vi "Bitfile.Initialize.vi"(8 "error in (no error)":errorcluster, 11 "FPGA Bitfile Settings":T1) -> (0 "error out":errorcluster, 3 "FPGA Session":u32)   [LabVIEW 2019, in "Diagnostics Addon Engine.lvlib"]
uses:
  Diagnostics Addon Engine.lvlib
  Addon Shared/Types/986x.ctl
  Addon Shared/Diagnostics Addon Shared.lvlib
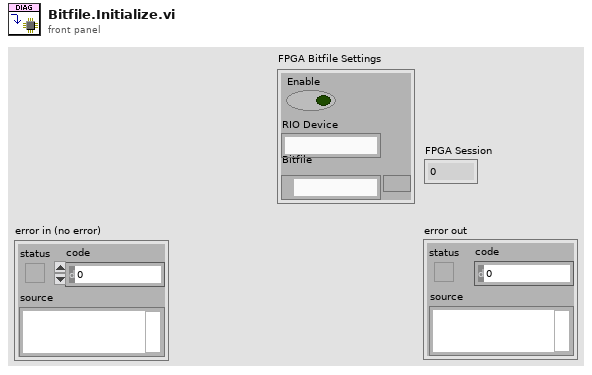
[diagram p1: front panel]
types:
  T1 = typedef "Diagnostics Addon Shared.lvlib/986x.ctl" = cluster{"Enable":bool, "RIO Device":string, "Bitfile":path}
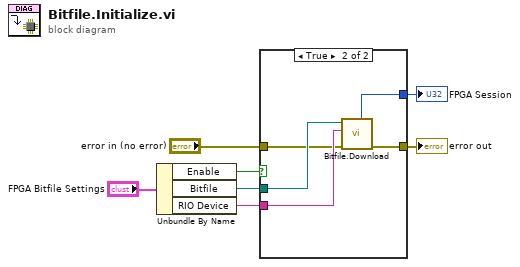
[diagram p0: block diagram]
diagram:
  n1 = Unbundle By Name("FPGA Bitfile Settings") -> ("Enable"=w3:bool, "Bitfile"=w2:path, "RIO Device"=w4:string)
  n2 = case shown="True" w3 {
    tunnel: "error in (no error)" -> [w8 w9]
    tunnel: [w8 w13] -> w7
    tunnel: [_ w12] -> w6
    tunnel: w4 -> [_ w11]
    tunnel: w2 -> [_ w10]
    frame False {
    }
    frame True {
      n3 = call "Bitfile.Download.vi"("error in (no error)"=w9, "Resource"=w11, "path"=w10) -> ("error out"=w13:errorcluster, "FPGA Session"=w12:u32)  [unwired: 7 in]
    }
  }
  "error out" <- w7
  "FPGA Session" <- w6
